vi "clearpath_set_differential_output.vi"(0 "ClearpathComm":T1, 1 "Right Output":dbl, 2 "Left Output":dbl) -> ()   [LabVIEW 2010, in "clearpath_interface.lvlib"]
doc: "Formats a Set Differential Setpoints command (0x202) to set the raw left and right motor output voltages as percentages of nominal (12V). Compensates for changes in battery voltages. Uses the onboard Clearpath library to perform the actual message formatting."
uses:
  clearpath_interface.lvlib
  cwrap_cRIO.dll
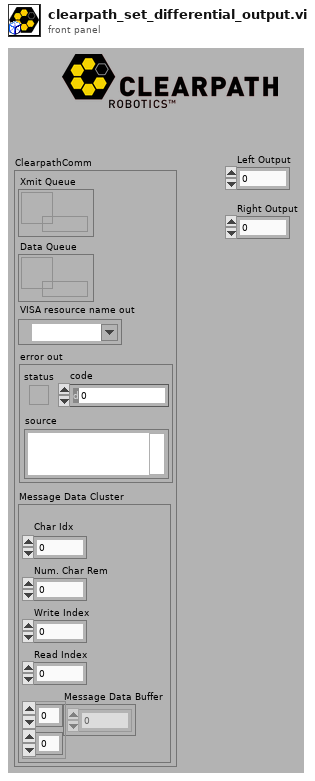
[diagram p1: front panel]
types:
  T1 = cluster{"Xmit Queue":refnum<queue>, "Data Queue":refnum<queue>, "VISA resource name out":refnum<visa-resource-name>, "error out":errorcluster, "Message Data Cluster":cluster{"\nChar Idx":u8, "Num. Char Rem":u8, "Write Index":u8, "Read Index":u8, "Message Data Buffer":u8[][]}}
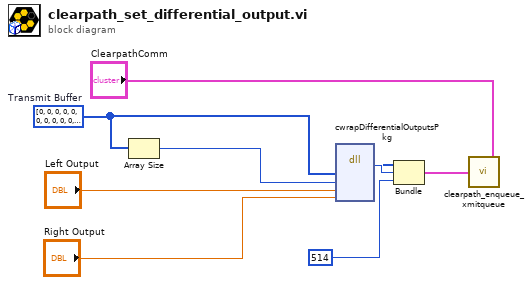
[diagram p0: block diagram]
diagram:
  w6 = u8[] [0, 0, 0, 0, 0, 0, 0, 0, 0, 0, 0, 0, 0, 0, 0, 0, 0, 0, 0, 0, 0, 0, 0, 0, 0, 0, 0, 0, 0, 0, 1, 0, 0, 0, 5]  # Transmit Buffer
  n1 = Array Size(array=w6) -> (size(s)=w7:i32)
  n2 = dll-call lib="cwrap_cRIO.*" fn="cwrapDifferentialOutputsPkg"("buf"=w6, "buf_size"=w7, "l_speed"="Left Output", "r_speed"="Right Output") -> ("return type"=w9:i32, "buf"=w8:u8[])  [unwired: 6 in, 2 out]
  n3 = Bundle("buf"=w8, "return type"=w9, 514) -> (w2:cluster{"buf":u8[], "return type":i32, i32})  [unwired: 1 in]
  n4 = call "clearpath_enqueue_xmitqueue.vi"("ClearpathComm"="ClearpathComm", "Cluster"=w2) -> ()
